vi "Populate Available Wfms.vi"(8 "error in":errorcluster, 9 "ListBox Variant":variant, 10 "CD Settings":T1={"CD Task Dependency"=18446744073709551615, "CD Task Dependency Ref"=18446744073709551615, "CD Task Available Wfms"=[], "CD Task Selected Wfms"=[], "Buffer Length (s)"=0.0, "Buffer Length (samples)"=0, "Single-point Enabled"=FALSE, "Running Average Enabled"=FALSE, "Task Rate"=0.0, "Scaled Waveform Enabled"=FALSE} {"CD Task Dependency Ref" format="%.0x"; "CD Task Dependency" format="%.0x"}, 11 "CustomDevice Ref":T2 format="%.0x") -> (0 "error out":errorcluster, 1 "ListBox Variant":variant, 2 "CD Settings out":T1={"CD Task Dependency"=18446744073709551615, "CD Task Dependency Ref"=18446744073709551615, "CD Task Available Wfms"=[], "CD Task Selected Wfms"=[], "Buffer Length (s)"=0.0, "Buffer Length (samples)"=0, "Single-point Enabled"=FALSE, "Running Average Enabled"=FALSE, "Task Rate"=0.0, "Scaled Waveform Enabled"=FALSE} {"CD Task Dependency Ref" format="%.0x"; "CD Task Dependency" format="%.0x"}, 3 "CustomDevice Ref":T2 format="%.0x")   [LabVIEW 2020, in "Waveform-Processing-Custom-Device System Explorer.lvlib"]
uses:
  Waveform-Processing-Custom-Device System Explorer.lvlib
  <vilib>/NI VeriStand/Custom Device API/Custom Device Item Ref.ctl
  Shared/Custom Device Settings.ctl
  NationalInstruments.VeriStand.SystemStorage
  NationalInstruments.VeriStand
  <vilib>/NI VeriStand/Custom Device Tools/Custom Device Utility Library/Custom Device Utility Library.lvlib
  <vilib>/NI VeriStand/Custom Device API/Custom Device API.lvlib
  Shared/Waveform-Processing-Custom-Device Shared.lvlib
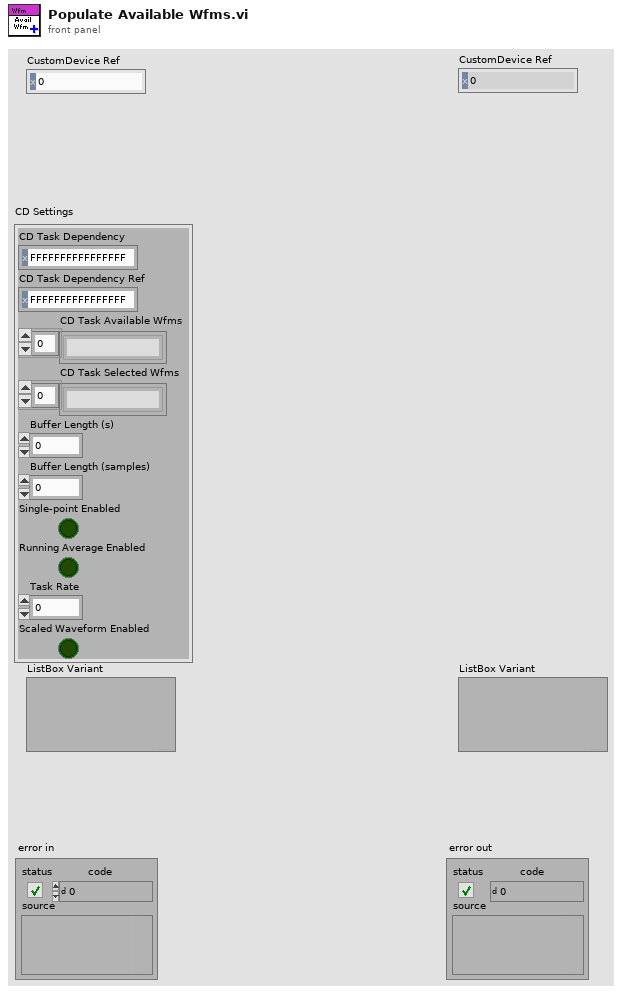
[diagram p1: front panel]
types:
  T1 = typedef "Waveform-Processing-Custom-Device Shared.lvlib/Custom Device Settings.ctl" = cluster{"CD Task Dependency":T2, "CD Task Dependency Ref":T2, "CD Task Available Wfms":string[], "CD Task Selected Wfms":string[], "Buffer Length (s)":dbl, "Buffer Length (samples)":u32, "Single-point Enabled":bool, "Running Average Enabled":bool, "Task Rate":dbl, "Scaled Waveform Enabled":bool}
  T2 = typedef "Custom Device API.lvlib/Custom Device Item Ref.ctl" = u64
  T3 = typedef "Custom Device API.lvlib/Custom Device Pointer.ctl" = refnum<k24>
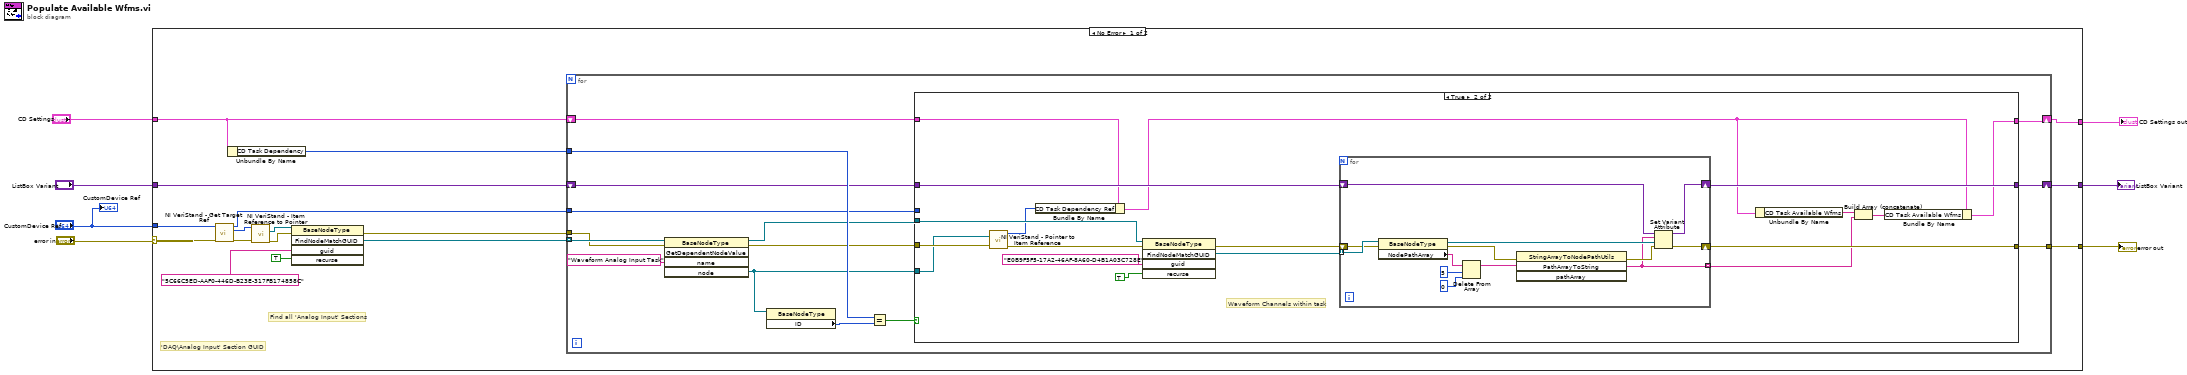
[diagram p0: block diagram]
diagram:
  n1 = case shown="No Error" "error in" {
    selector: "error in" -> [w24 w76]
    tunnel: [w16 w76] -> w4
    tunnel: "CustomDevice Ref" -> [w13 _]
    tunnel: [w15 w75] -> w5
    tunnel: "ListBox Variant" -> [w14 w75]
    tunnel: "CD Settings" -> [w10 w74]
    tunnel: [w9 w74] -> w1
    frame No Error {
      # "'DAQ\\Analog Input' Section GUID"
      # "Find all 'Analog Input' Sections"
      n2 = call <vilib>:"NI VeriStand - Get Target Ref.vi"("error in"=w24, "Item Ref in"=w13) -> ("error out"=w23:errorcluster, "Target Ref"=w22:T2, "Item Ref out"=w12:T2)  [unwired: 6 in, 1 out]
      n3 = Unbundle By Name(w10) -> ("CD Task Dependency"=w11:T2)
      n4 = call <vilib>:"NI VeriStand - Item Reference to Pointer.vi"("error in (no error)"=w23, "Item Ref in"=w22) -> ("error out"=w20:errorcluster, "Node Pointer"=w21:T3)  [unwired: 6 in, 2 out]
      n5 = invoke class="BaseNodeType" method="FindNodeMatchGUID"(reference=w21, error in=w20, "guid"="5C66C5ED-AAF0-446D-B23E-317FB174858C" ("Item GUID"), "recurse"=TRUE ("Find All? (T)")) -> (error out=w17:errorcluster, "FindNodeMatchGUID"=w8:refnum<k24>[])  [unwired: 1 in, 3 out]
      n6 = for {
        tunnel: w11 -> [w39]
        tunnel: w8 -> [w38] mode=indexing
        tunnel: w17 -> [w37]
        tunnel: [w32] -> w16
        shift-right: [w31] -> w15
        shift-left: w14 -> [w30]
        tunnel: w12 -> [w29]
        shift-right: [w25] -> w9
        shift-left: w10 -> [w26]
        n7 = invoke class="BaseNodeType" method="GetDependentNodeValue"(reference=w38, error in=w37, "name"="Waveform Analog Input Task" ("Property Name")) -> (reference out=w27:refnum<k24>, error out=w34:errorcluster, "node"=w28:refnum<k24>)  [unwired: 2 in, 2 out]
        n8 = property class="BaseNodeType"(reference=w28) -> ("ID"=w35:u64)  [unwired: 1 in, 2 out]
        n9 = Equal?(x=w39, y=w35) -> (x = y?=w33:bool)
        n10 = case shown="True" w33 {
          tunnel: w28 -> [_ w52]
          tunnel: w34 -> [w42 w53]
          tunnel: [w42 w56] -> w32
          tunnel: [w41 w55] -> w31
          tunnel: w30 -> [w41 w54]
          tunnel: w29 -> [_ _]
          tunnel: w27 -> [_ w51]
          tunnel: w26 -> [w40 w50]
          tunnel: [w40 w43] -> w25
          frame False {
          }
          frame True {
            # "Waveform Channels within task"
            n11 = call <vilib>:"NI VeriStand - Pointer to Item Reference.vi"("error in (no error)"=w53, "Node Pointer"=w52) -> ("error out"=w48:errorcluster, "Item Ref out"=w49:T2)  [unwired: 8 in]
            n12 = Bundle By Name(cluster=w50, "CD Task Dependency Ref"=w49) -> (w45:T1)
            n13 = invoke class="BaseNodeType" method="FindNodeMatchGUID"(reference=w51, error in=w48, "guid"="E0B9F5F5-17A2-46AF-8A60-D4B1A03C728E", "recurse"=TRUE ("Find All? (T)")) -> (error out=w57:errorcluster, "FindNodeMatchGUID"=w58:refnum<k24>[])  [unwired: 1 in, 3 out]
            n14 = for {
              tunnel: w58 -> [w69] mode=indexing
              shift-right: [w65] -> w55
              shift-left: w54 -> [w64]
              shift-right: [w66] -> w56
              shift-left: w57 -> [w68]
              tunnel: [w61] -> w46 mode=indexing
              n15 = property class="BaseNodeType"(reference=w69, error in=w68) -> (reference out=w63:refnum<k24>, error out=w67:errorcluster, "NodePathArray"=w70:string[])
              n16 = Delete From Array(array=w70, length=5, index=0) -> (array with subset deleted=w73:string[])  [unwired: 1 out]
              n17 = invoke class="StringArrayToNodePathUtils" method="PathArrayToString"(error in=w67, "pathArray"=w73) -> (error out=w62:errorcluster, "PathArrayToString"=w61:string)  [unwired: 2 in, 2 out]
              n18 = Set Variant Attribute(Variant=w64, name=w61, value=w63, error in=w62) -> (Variant out=w65:variant, error out=w66:errorcluster)  [unwired: 1 out]
            }
            n19 = Unbundle By Name(w45) -> ("CD Task Available Wfms"=w47:string[])
            n20 = Build Array (concatenate)(w47, w46) -> (w44:string[])
            n21 = Bundle By Name(cluster=w45, "CD Task Available Wfms"=w44) -> (w43:T1)
          }
        }
      }
    }
    frame Error {
    }
  }
  "error out" <- w4
  "ListBox Variant" <- w5
  "CD Settings out" <- w1
  "CustomDevice Ref" <- "CustomDevice Ref"
